vi "AOTFSettings.vi"(1 "Get/Set":bool, 2 "AOTF Setting (Input)":T1={"Laser 1 Output Channel"="0", "AOTF  1 Output Voltage"=5.0, "Laser 2 Output Channel"="1", "AOTF  2 Output Voltage"=5.0, "Laser 3 Output Channel"="2", "AOTF  3 Output Voltage"=5.0, "Pixel per Cycle"=3, "Time per Cycle  / ms"=0.1, "Laser 4 Output Channel"="3", "AOTF  4 Output Voltage"=5.0, "Laser 5 Output Channel"="4", "AOTF 5 Output Voltage "=5.0, "Laser 6 Output Channel"="5", "AOTF  6 Output Voltage "=5.0, "Laser 7 Output Channel"="6", "AOTF 7 Output Voltage "=5.0, "Laser 8 Output Channel"="7", "AOTF  8 Output Voltage "=5.0, "AOTF  1 Frequency"=90.6, "AOTF  2 Frequency"=94.6, "AOTF  3  Frequency"=99.8, "AOTF  4 Frequency"=105.3, "AOTF 5 Frequency"=111.6, "AOTF  6 Frequency"=118.8, "AOTF 7  Frequency"=127.4, "AOTF  8 Frequency"=137.0, "AOTF  1 Amplitude"=13000.0, "AOTF  2 Amplitude"=13000.0, "AOTF  3  Amplitude"=13000.0, "AOTF  4 Amplitude"=13000.0, "AOTF 5 Amplitude"=14000.0, "AOTF  6 Amplitude"=14000.0, "AOTF 7 Amplitude  "=14000.0, "AOTF  8 Amplitude"=14000.0} {"AOTF  8 Amplitude" format="%.2f"; "AOTF 7 Amplitude" format="%.2f"; "AOTF  6 Amplitude" format="%.2f"; "AOTF 5 Amplitude" format="%.2f"; "AOTF  4 Amplitude" format="%.2f"; "AOTF  3  Amplitude" min=0.0 max=10000000.0 format="%.2f"; "AOTF  2 Amplitude" min=0.0 max=10000000.0 format="%.2f"; "AOTF  1 Amplitude" min=0.0 max=1000000.0 format="%.2f"; "AOTF  8 Frequency" format="%.2f"; "AOTF 7  Frequency" format="%.2f"; "AOTF  6 Frequency" format="%.2f"; "AOTF 5 Frequency" format="%.2f"; "AOTF  4 Frequency" format="%.2f"; "AOTF  3  Frequency" min=0.0 max=10000000.0 format="%.2f"; "AOTF  2 Frequency" min=0.0 max=10000000.0 format="%.2f"; "AOTF  1 Frequency" min=0.0 max=1000000.0 format="%.2f"; "AOTF  8 Output Voltage" format="%.2f"; "AOTF 7 Output Voltage" format="%.2f"; "AOTF  6 Output Voltage" format="%.2f"; "AOTF 5 Output Voltage" format="%.2f"; "AOTF  4 Output Voltage" format="%.2f"; "Time per Cycle  / ms" format="%#.3f"; "AOTF  3 Output Voltage" format="%.2f"; "AOTF  2 Output Voltage" format="%.2f"; "AOTF  1 Output Voltage" format="%.2f"}) -> (0 "AOTF Setting (Output)":T1={"Laser 1 Output Channel"="5", "AOTF  1 Output Voltage"=5.0, "Laser 2 Output Channel"="6", "AOTF  2 Output Voltage"=5.0, "Laser 3 Output Channel"="1", "AOTF  3 Output Voltage"=0.0, "Pixel per Cycle"=3, "Time per Cycle  / ms"=0.1, "Laser 4 Output Channel"="1", "AOTF  4 Output Voltage"=0.0, "Laser 5 Output Channel"="1", "AOTF 5 Output Voltage "=0.0, "Laser 6 Output Channel"="1", "AOTF  6 Output Voltage "=0.0, "Laser 7 Output Channel"="1", "AOTF 7 Output Voltage "=0.0, "Laser 8 Output Channel"="1", "AOTF  8 Output Voltage "=0.0, "AOTF  1 Frequency"=840000.0, "AOTF  2 Frequency"=880000.0, "AOTF  3  Frequency"=940000.0, "AOTF  4 Frequency"=1010000.0, "AOTF 5 Frequency"=1090000.0, "AOTF  6 Frequency"=1190000.0, "AOTF 7  Frequency"=1270000.0, "AOTF  8 Frequency"=1370000.0, "AOTF  1 Amplitude"=84.0, "AOTF  2 Amplitude"=88.0, "AOTF  3  Amplitude"=94.0, "AOTF  4 Amplitude"=101.0, "AOTF 5 Amplitude"=109.0, "AOTF  6 Amplitude"=119.0, "AOTF 7 Amplitude  "=127.0, "AOTF  8 Amplitude"=137.0} {"AOTF  8 Amplitude" format="%.2f"; "AOTF 7 Amplitude" format="%.2f"; "AOTF  6 Amplitude" format="%.2f"; "AOTF 5 Amplitude" format="%.2f"; "AOTF  4 Amplitude" format="%.2f"; "AOTF  3  Amplitude" min=0.0 max=10000000.0 format="%.2f"; "AOTF  2 Amplitude" min=0.0 max=10000000.0 format="%.2f"; "AOTF  1 Amplitude" min=0.0 max=1000000.0 format="%.2f"; "AOTF  8 Frequency" format="%.2f"; "AOTF 7  Frequency" format="%.2f"; "AOTF  6 Frequency" format="%.2f"; "AOTF 5 Frequency" format="%.2f"; "AOTF  4 Frequency" format="%.2f"; "AOTF  3  Frequency" min=0.0 max=10000000.0 format="%.2f"; "AOTF  2 Frequency" min=0.0 max=10000000.0 format="%.2f"; "AOTF  1 Frequency" min=0.0 max=1000000.0 format="%.2f"; "AOTF  8 Output Voltage" format="%.2f"; "AOTF 7 Output Voltage" format="%.2f"; "AOTF  6 Output Voltage" format="%.2f"; "AOTF 5 Output Voltage" format="%.2f"; "AOTF  4 Output Voltage" format="%.2f"; "Time per Cycle  / ms" format="%#.3f"; "AOTF  3 Output Voltage" format="%.2f"; "AOTF  2 Output Voltage" format="%.2f"; "AOTF  1 Output Voltage" format="%.2f"})   [LabVIEW 2009]
uses:
  AOTFSettings.ctt
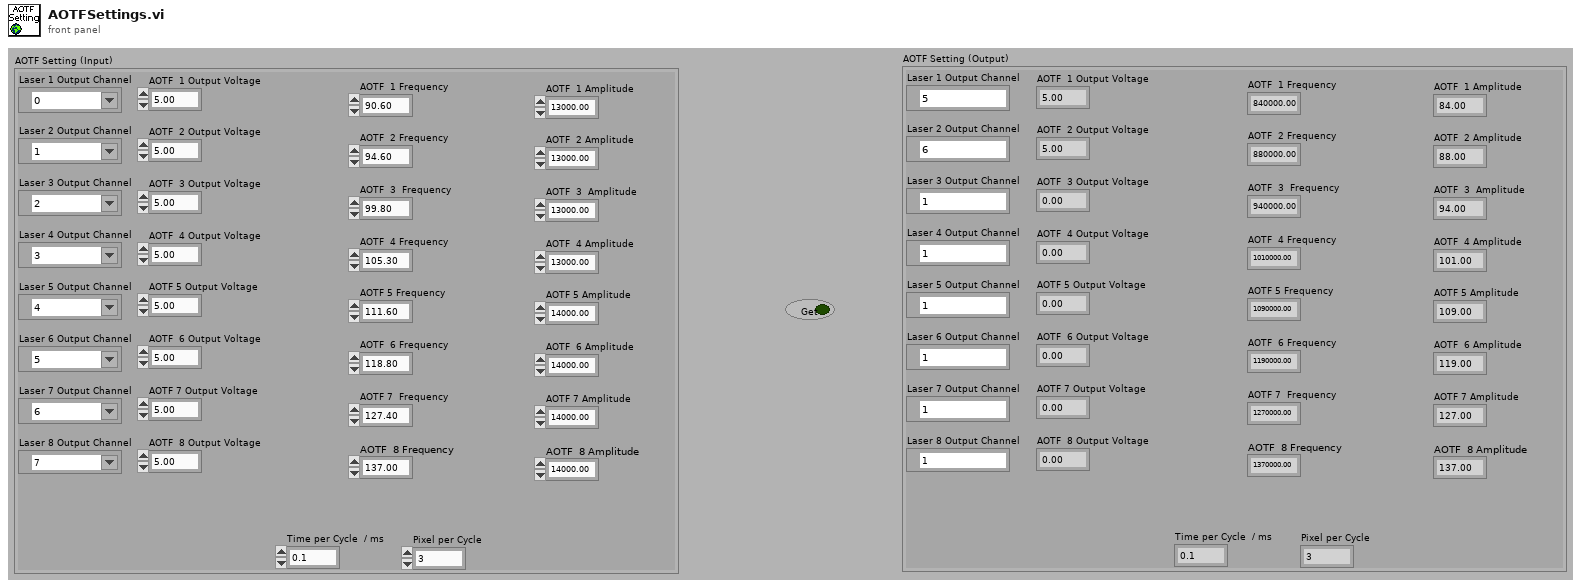
[diagram p1: front panel]
types:
  T1 = typedef "AOTFSettings.ctt" = cluster{"Laser 1 Output Channel":tag, "AOTF  1 Output Voltage":dbl, "Laser 2 Output Channel":tag, "AOTF  2 Output Voltage":dbl, "Laser 3 Output Channel":tag, "AOTF  3 Output Voltage":dbl, "Pixel per Cycle":u16, "Time per Cycle  / ms":dbl, "Laser 4 Output Channel":tag, "AOTF  4 Output Voltage":dbl, "Laser 5 Output Channel":tag, "AOTF 5 Output Voltage ":dbl, "Laser 6 Output Channel":tag, "AOTF  6 Output Voltage ":dbl, "Laser 7 Output Channel":tag, "AOTF 7 Output Voltage ":dbl, "Laser 8 Output Channel":tag, "AOTF  8 Output Voltage ":dbl, "AOTF  1 Frequency":dbl, "AOTF  2 Frequency":dbl, "AOTF  3  Frequency":dbl, "AOTF  4 Frequency":dbl, "AOTF 5 Frequency":dbl, "AOTF  6 Frequency":dbl, "AOTF 7  Frequency":dbl, "AOTF  8 Frequency":dbl, "AOTF  1 Amplitude":dbl, "AOTF  2 Amplitude":dbl, "AOTF  3  Amplitude":dbl, "AOTF  4 Amplitude":dbl, "AOTF 5 Amplitude":dbl, "AOTF  6 Amplitude":dbl, "AOTF 7 Amplitude  ":dbl, "AOTF  8 Amplitude":dbl}
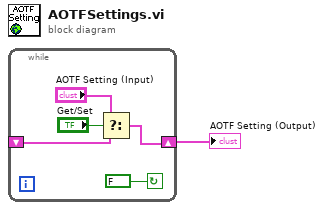
[diagram p0: block diagram]
diagram:
  n1 = while {
    shift-right: [w2] -> w1
    shift-left: _ -> [w5]
    stop <- FALSE continue-if-true
    n2 = Select(t="AOTF Setting (Input)", s="Get/Set", f=w5) -> (s? t:f=w2:T1)
  }
  "AOTF Setting (Output)" <- w1
